vi "appSupportFolderPath.vi"() -> (15 "Support path":path)   [LabVIEW 2022 SP3, in "stillnessHelper.lvclass"]
doc: "This vi returns the \"support\" folder of the application. So in the development environment it send back the \"project\" support sub-folder and if it is a compiled version, it send the software installation support sub-folder!"
uses:
  stillnessHelper.lvclass
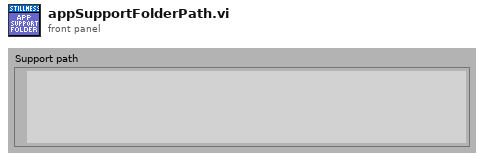
[diagram p1: front panel]
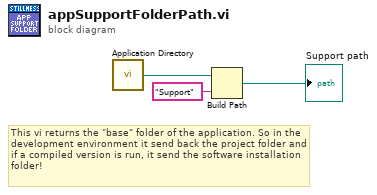
[diagram p0: block diagram]
diagram:
  # "This vi returns the \"base\" folder of the application. So in the development environment it send back the project folder and if a compiled version is run, it send the software installation folder!"
  n1 = call <vilib>:"Application Directory.vi"() -> ("Application Directory"=w3:path)
  n2 = Build Path(base path=w3, name or relative path="Support") -> (appended path=→"Support path":path)
